vi "Configure Protection Limits.vi"(6 "Low Voltage Limit (0)":dbl, 7 "Over Current Protection Detection Time (0 S)":dbl, 8 "error in (no error)":errorcluster, 9 "Overvoltage Protection Limit (0)":dbl, 10 "Overcurrent Protection Limit (0)":dbl, 11 "VISA resource name":refnum<visa-resource-name>) -> (0 "error out":errorcluster, 3 "VISA resource name out":refnum<visa-resource-name>)   [LabVIEW 2023]
doc: "Configures the overvoltage and overcurrent protection limits."
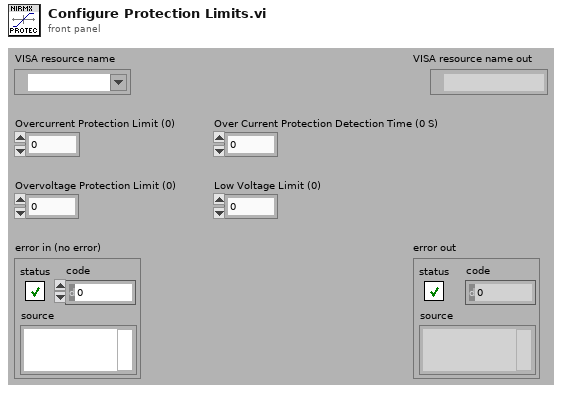
[diagram p1: front panel]
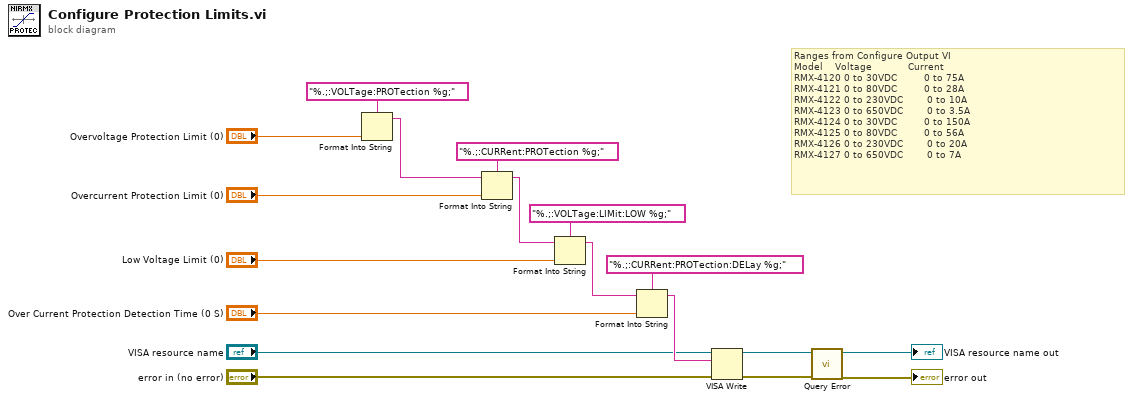
[diagram p0: block diagram]
diagram:
  # "Ranges from Configure Output VI\nModel    Voltage            Current\nRMX-4120\t0 to 30VDC\t        0 to 75A\nRMX-4121\t0 to 80VDC\t        0 to 28A\nRMX-4122\t0 to 230VDC\t       0 to 10A\nRMX-4123\t0 to 650VDC\t       0 to 3.5A\nRMX-4124\t0 to 30VDC\t        0 to 150A\nRMX-4125\t0 to 80VDC\t        0 to 56A\nRMX-4126\t0 to 230VDC\t       0 to 20A\nRMX-4127\t0 to 650VDC\t       0 to 7A"
  n1 = Format Into String(format string="%.;:VOLTage:PROTection %g;", "Overvoltage Protection Limit (0)") -> (resulting string=w16:string)  [unwired: 2 in, 1 out]
  n2 = Format Into String(format string="%.;:CURRent:PROTection %g;", initial string=w16, "Overcurrent Protection Limit (0)") -> (resulting string=w3:string)  [unwired: 1 in, 1 out]
  n3 = Format Into String(format string="%.;:VOLTage:LIMit:LOW %g;", initial string=w3, "Low Voltage Limit (0)") -> (resulting string=w2:string)  [unwired: 1 in, 1 out]
  n4 = Format Into String(format string="%.;:CURRent:PROTection:DELay %g;", initial string=w2, "Over Current Protection Detection Time (0 S)") -> (resulting string=w11:string)  [unwired: 1 in, 1 out]
  n5 = VISA Write(VISA resource name="VISA resource name", write buffer=w11, error in (no error)="error in (no error)") -> (VISA resource name out=w8:refnum<visa-resource-name>, error out=w7:errorcluster)  [unwired: 1 out]
  n6 = call "Query Error.vi"("error in (no error)"=w7, "VISA resource name"=w8) -> ("error out"=→"error out":errorcluster, "VISA resource name out"=→"VISA resource name out":refnum<visa-resource-name>)  [unwired: 6 in, 2 out]
